vi "Smart IO Set Pwm Output.vi"(8 "error in (no error)":errorcluster, 10 "value (-1 to 1)":dbl, 11 "deviceIndex":i32) -> (0 "error out":errorcluster)   [LabVIEW 2026, in "MrcLib.lvlib"]
doc: "Set the PWM output value. Motors, servos???"
uses:
  MrcLib.lvlib
  Types/MRC Smart IO Mode.ctl
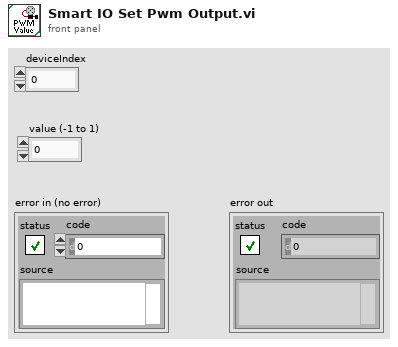
[diagram p1: front panel]
types:
  T1 = typedef "MRC Smart IO Mode.ctl" = i32
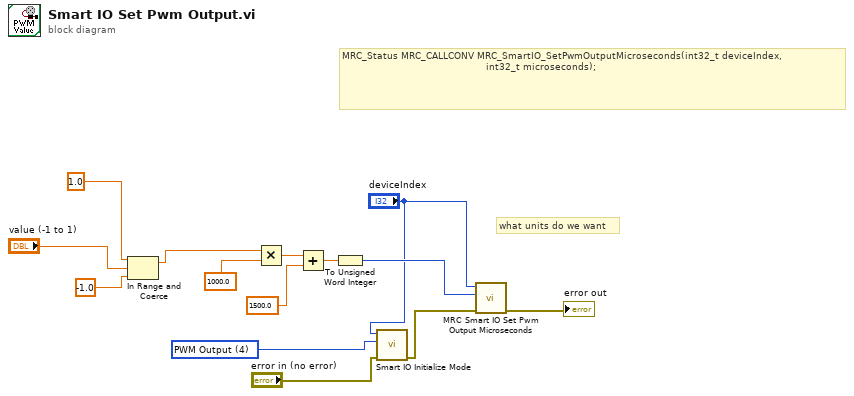
[diagram p0: block diagram]
diagram:
  w1 = T1 4 items=["Digital Input"=0, "Digital Output"=1, "Analog Input"=2, "PWM Input"=3, "PWM Output"=4, "Counter Rising"=5, "Counter Falling"=6, "Addressable LEDs"=13] ("mode")
  # "what units do we want"
  # "MRC_Status MRC_CALLCONV MRC_SmartIO_SetPwmOutputMicroseconds(int32_t deviceIndex,\n                                                int32_t microseconds);"
  n1 = In Range and Coerce(upper limit=1.0, x="value (-1 to 1)", lower limit=-1.0) -> (coerced(x)=w9:dbl)  [unwired: 1 out]
  n2 = Multiply(x=w9, y=1000.0) -> (x*y=w12:dbl)
  n3 = Add(x=w12, y=1500.0) -> (x+y=w6:dbl)
  n4 = To Unsigned Word Integer(number=w6) -> (unsigned 16bit integer=w5:u16)
  n5 = call "Smart IO Initialize Mode.vi"("error in (no error)"="error in (no error)", "mode"=w1, "deviceIndex"="deviceIndex") -> ("error out"=w4:errorcluster)  [unwired: 8 in]
  n6 = call "MRC Smart IO Set Pwm Output Microseconds.vi"("error in (no error)"=w4, "microseconds"=w5, "deviceIndex"="deviceIndex") -> ("error out"=→"error out":errorcluster)  [unwired: 8 in]
